vi "OpenImageFile.vi"(3 "selected path":path) -> (1 "Image Out":T1 {"Dialogs" format="%.0b"})   [LabVIEW 2024]
doc: "This VI will load an image from your hard disk or some other specified source."
uses:
  <userlib>/ImageProcessing/QTLIB_2595_LV86/QT_Image.ctl
  <vilib>/picture/picture.llb/imagedata.ctl
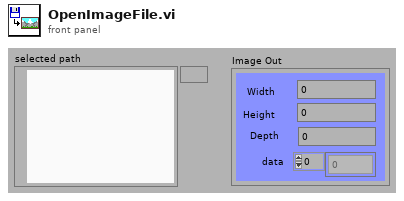
[diagram p1: front panel]
types:
  T1 = typedef "QT_Image.ctl" = cluster{"Width":i32, "Height":i32, "Depth":i32, "data":u8[], "Compressed data":u8[], "Color table":u32[], "Duration":i32, "Options":i32, "Timestamp":i32, "ID":i32, "Reserved":i32, "Dialogs":u32}
  T2 = typedef "imagedata.ctl" = cluster{"image type":i32, "image depth":i32, "image":u8[], "mask":u8[], "colors":u32[], "Rectangle":cluster{"left":i16, "top":i16, "right":i16, "bottom":i16}}
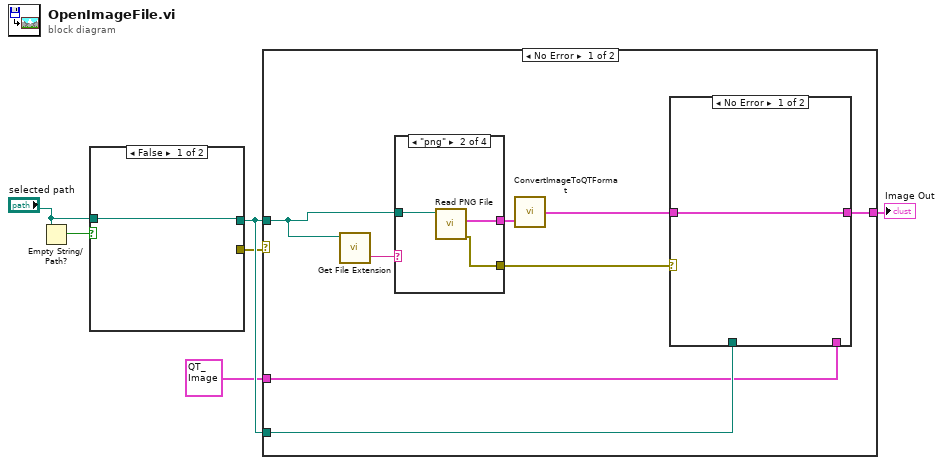
[diagram p0: block diagram]
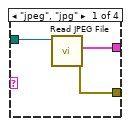
[diagram p2: hidden frame]
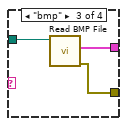
[diagram p3: hidden frame]
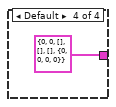
[diagram p4: hidden frame]
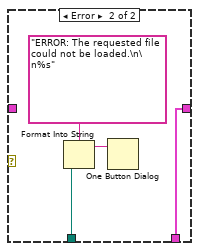
[diagram p5: hidden frame]
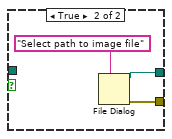
[diagram p7: hidden frame]
diagram:
  n1 = Empty String/Path?(string/path="selected path") -> (empty?=w5:bool)
  n2 = case shown="False" w5 {
    tunnel: [w7 w10] -> w6
    tunnel: "selected path" -> [w7 _]
    tunnel: [_ w9] -> w3
    frame False {
    }
    frame True {
      n3 = File Dialog(7:"Select path to image file" ("prompt")) -> (0:w9:errorcluster, 3:w10:path)  [unwired: 1 in, 7 out]
    }
  }
  n4 = case shown="No Error" w3 {
    tunnel: w6 -> [w12 _]
    tunnel: w6 -> [w17 _]
    tunnel: [w16 w34] -> w2
    tunnel: T1 {"Width"=378, "Height"=255, "Depth"=24, "data"=array[289170 elements], "Compressed data"=[], "Color table"=[], "Duration"=0, "Options"=0, "Timestamp"=0, "ID"=0, "Reserved"=0, "Dialogs"=0} ("Image Out 2") -> [w14 w34]
    frame No Error {
      n5 = call <vilib>:"Get File Extension.vi"("file"=w12) -> ("unmodified file extension"=w11:string)  [unwired: 6 in, 4 out]
      n6 = case shown="\"png\"" w11 {
        tunnel: w12 -> [w21 w24 w27 _]
        tunnel: [w20 w23 w26 T2 {"image type"=0, "image depth"=0, "image"=[], "mask"=[], "colors"=[], "Rectangle"={"left"=0, "top"=0, "right"=0, "bottom"=0}} ("image data")] -> w13
        tunnel: [w19 w22 w25 _] -> w18
        frame "jpeg", "jpg" {
          n7 = call <vilib>:"Read JPEG File.vi"("path to JPEG file"=w21) -> ("error out"=w19:errorcluster, "image data"=w20:T2)  [unwired: 8 in, 1 out]
        }
        frame "png" {
          n8 = call <vilib>:"Read PNG File.vi"("path to PNG file"=w24) -> ("error out"=w22:errorcluster, "image data"=w23:T2)  [unwired: 8 in, 1 out]
        }
        frame "bmp" {
          n9 = call <vilib>:"Read BMP File.vi"("path to BMP file"=w27) -> ("error out"=w25:errorcluster, "image data"=w26:T2)  [unwired: 8 in, 1 out]
        }
        frame Default {
        }
      }
      n10 = call <userlib>:"ConvertImageToQTFormat.vi"("image data"=w13) -> ("Image Out"=w15:T1)
      n11 = case shown="No Error" w18 {
        tunnel: w17 -> [_ w32]
        tunnel: [w29 w30] -> w16
        tunnel: w15 -> [w29 _]
        tunnel: w14 -> [_ w30]
        frame No Error {
        }
        frame Error {
          n12 = Format Into String(format string="ERROR: The requested file could not be loaded.\n\n%s" ("Path"), w32) -> (resulting string=w31:string)  [unwired: 2 in, 1 out]
          n13 = One Button Dialog(message=w31) -> ()  [unwired: 1 in, 1 out]
        }
      }
    }
    frame Error {
    }
  }
  "Image Out" <- w2
